vi "JOG.vi"(2 "baud rate (9600)":u32=115200 caption="보 전송속도(9600)", 3 "AXIS":u16(ring) items=["+X", "-X", "+Y", "-Y"], 4 "Port":refnum<visa-resource-name>="COM4" caption="VISA 리소스 이름") -> (0 "Error Out":errorcluster caption="에러 출력", 1 "VISA out":refnum<visa-resource-name>)   [LabVIEW 2016]
uses:
  <vilib>/Instr/_visa.llb/VISA Configure Serial Port (Instr).vi
  <vilib>/Instr/_visa.llb/VISA Flush IO Buffer Mask.ctl
panel:
  out "Commend Count":u32
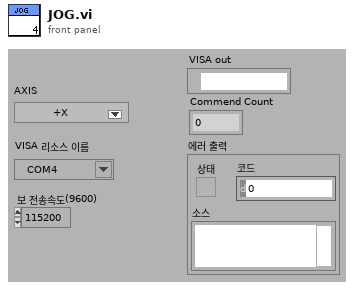
[diagram p1: front panel]
types:
  T1 = typedef "VISA Flush IO Buffer Mask.ctl" = u16
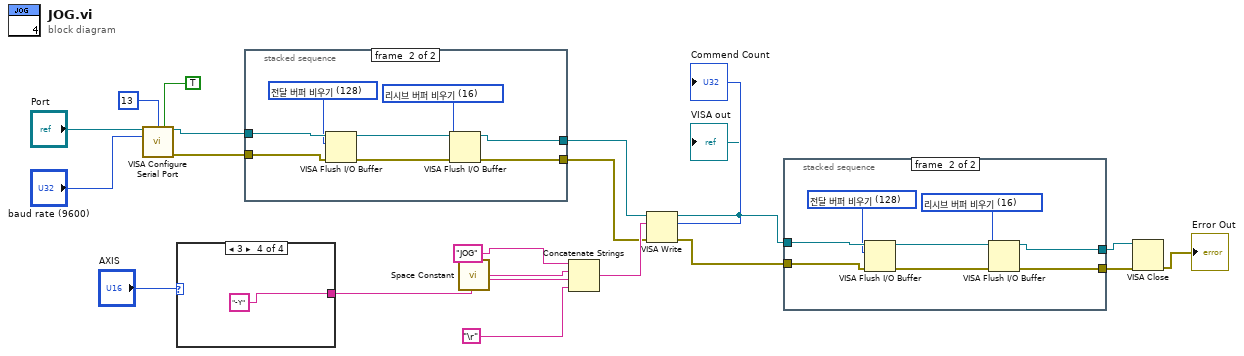
[diagram p0: block diagram]
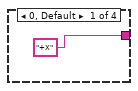
[diagram p2: hidden frame]
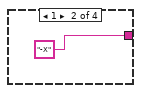
[diagram p3: hidden frame]
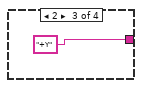
[diagram p4: hidden frame]
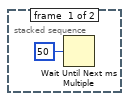
[diagram p5: hidden frame]
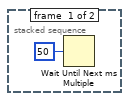
[diagram p6: hidden frame]
diagram:
  n1 = call-poly "VISA Configure Serial Port"("VISA resource name"="Port", "termination char\n(0xA = '\\n' = LF)"=i16 13 ("termination char\n(0xA = '\\n' = LF)"), "Enable Termination\nChar (T)"=TRUE ("Enable Termination\nChar (T)"), "baud rate (9600)"="baud rate (9600)") -> ("VISA resource name out"=w11:refnum<visa-resource-name>, "error out"=w10:errorcluster)  [unwired: 10 in]
  n2 = case shown="3" "AXIS" {
    tunnel: ["+X" "-X" "+Y" "-Y"] -> w1
    frame 0, Default {
    }
    frame 1 {
    }
    frame 2 {
    }
    frame 3 {
    }
  }
  n3 = stacked-sequence {
    tunnel: w11 -> [_ w33]
    tunnel: w10 -> [_ w32]
    tunnel: [_ w28] -> w4
    tunnel: [_ w27] -> w3
    frame #0 {
      n4 = Wait Until Next ms Multiple(millisecond multiple=u32 50 ("ms 배수")) -> ()  [unwired: 1 out]
    }
    frame #1 {
      w26 = T1 16 items=["리시브 버퍼 비우기"=16, "전달 버퍼 디바이스에 쓰기"=32, "리시브 버퍼 비우기(I/O 없음)"=64, "전달 버퍼 비우기"=128] ("Mask")
      w31 = T1 128 items=["리시브 버퍼 비우기"=16, "전달 버퍼 디바이스에 쓰기"=32, "리시브 버퍼 비우기(I/O 없음)"=64, "전달 버퍼 비우기"=128] ("Mask")
      n5 = VISA Flush I/O Buffer(VISA resource name=w33, mask (16)=w31, error in (no error)=w32) -> (VISA resource name out=w30:refnum<visa-resource-name>, error out=w29:errorcluster)
      n6 = VISA Flush I/O Buffer(VISA resource name=w30, mask (16)=w26, error in (no error)=w29) -> (VISA resource name out=w28:refnum<visa-resource-name>, error out=w27:errorcluster)
    }
  }
  n7 = call <vilib>:"Space Constant.vi"() -> ("String"=w19:string)
  n8 = Concatenate Strings("JOG", w19, w1, "\r") -> (w17:string)
  n9 = VISA Write(VISA resource name=w4, write buffer=w17, error in (no error)=w3) -> (VISA resource name out=w6:refnum<visa-resource-name>, return count=→"Commend Count":u32, error out=w5:errorcluster)
  "VISA out" <- w6
  n10 = stacked-sequence {
    tunnel: w6 -> [_ w42]
    tunnel: w5 -> [_ w41]
    tunnel: [_ w37] -> w8
    tunnel: [_ w36] -> w9
    frame #0 {
      n11 = Wait Until Next ms Multiple(millisecond multiple=u32 50 ("ms 배수")) -> ()  [unwired: 1 out]
    }
    frame #1 {
      w35 = T1 16 items=["리시브 버퍼 비우기"=16, "전달 버퍼 디바이스에 쓰기"=32, "리시브 버퍼 비우기(I/O 없음)"=64, "전달 버퍼 비우기"=128] ("Mask")
      w40 = T1 128 items=["리시브 버퍼 비우기"=16, "전달 버퍼 디바이스에 쓰기"=32, "리시브 버퍼 비우기(I/O 없음)"=64, "전달 버퍼 비우기"=128] ("Mask")
      n12 = VISA Flush I/O Buffer(VISA resource name=w42, mask (16)=w40, error in (no error)=w41) -> (VISA resource name out=w39:refnum<visa-resource-name>, error out=w38:errorcluster)
      n13 = VISA Flush I/O Buffer(VISA resource name=w39, mask (16)=w35, error in (no error)=w38) -> (VISA resource name out=w37:refnum<visa-resource-name>, error out=w36:errorcluster)
    }
  }
  n14 = VISA Close(VISA resource name=w8, error in (no error)=w9) -> (error out=→"Error Out":errorcluster)
